vi "VMI_delays_combine.vi"(0 "Peak Array All":cluster{"X":sgl, "Y":sgl}[][][](array[cluster]), 4 "AI per delay All":dbl[][][](array[numeric]), 5 "Peak Array Current":cluster{"X":sgl, "Y":sgl}[][][](array[cluster]), 6 "AI per delay Current":dbl[][][](array[numeric]), 7 "Delay Number":i32, 9 "Counts per delay All":dbl[][][](array[numeric]), 10 "Std per delay All":dbl[][][](array[numeric]), 11 "Counts per delay Current":dbl[][][](array[numeric]), 15 "Std per delay Current":dbl[][][](array[numeric])) -> (1 "Peak Out":cluster{"X":sgl, "Y":sgl}[][][](array[cluster]), 3 "AI Out":dbl[][][](array[numeric]), 12 "Counts Out":dbl[][][](array[numeric]), 14 "Std Out":dbl[][][](array[numeric]))   [LabVIEW 2020]
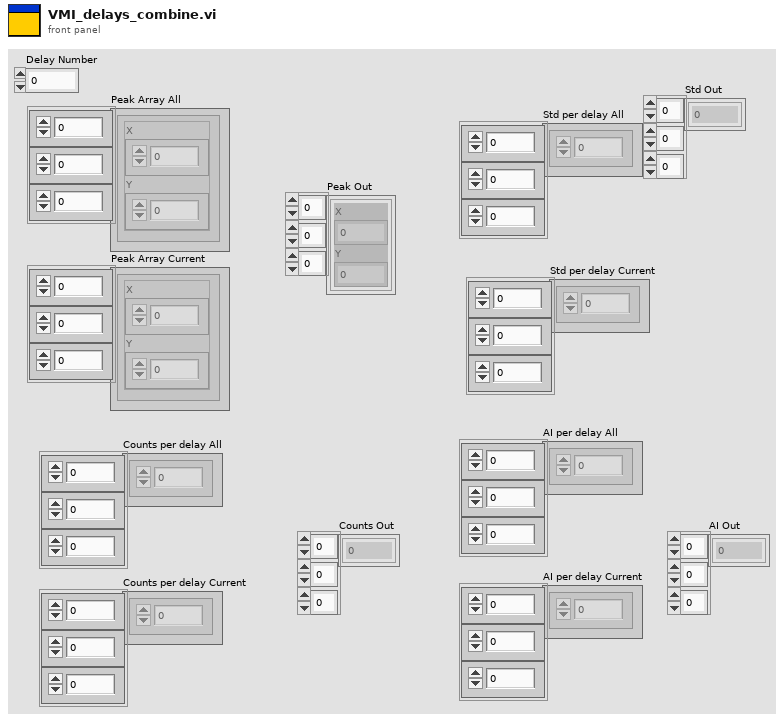
[diagram p1: front panel]
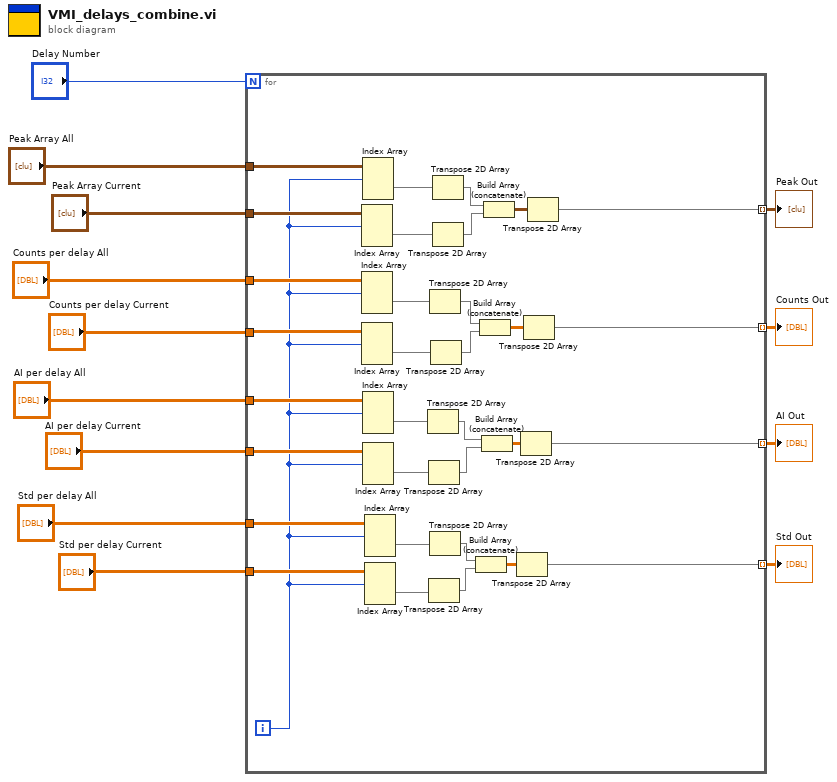
[diagram p0: block diagram]
diagram:
  n1 = for {
    N: "Delay Number" -> [_]
    tunnel: "Peak Array All" -> [w46]
    tunnel: "Counts per delay All" -> [w45]
    tunnel: "AI per delay All" -> [w44]
    tunnel: "Std per delay All" -> [w43]
    tunnel: "Peak Array Current" -> [w41]
    tunnel: [w36] -> w7 mode=indexing
    tunnel: "Counts per delay Current" -> [w34]
    tunnel: [w29] -> w5 mode=indexing
    tunnel: "AI per delay Current" -> [w28]
    tunnel: [w22] -> w3 mode=indexing
    tunnel: "Std per delay Current" -> [w21]
    tunnel: [w14] -> w1 mode=indexing
    i -> [w20]
    n2 = Index Array(array=w41, index (dim 0)=w20) -> (element=w40:cluster{"X":sgl, "Y":sgl}[][])  [unwired: 2 in]
    n3 = Index Array(array=w45, index (dim 0)=w20) -> (element=w35:dbl[][])  [unwired: 2 in]
    n4 = Index Array(array=w34, index (dim 0)=w20) -> (element=w33:dbl[][])  [unwired: 2 in]
    n5 = Index Array(array=w46, index (dim 0)=w20) -> (element=w42:cluster{"X":sgl, "Y":sgl}[][])  [unwired: 2 in]
    n6 = Index Array(array=w44, index (dim 0)=w20) -> (element=w27:dbl[][])  [unwired: 2 in]
    n7 = Index Array(array=w28, index (dim 0)=w20) -> (element=w26:dbl[][])  [unwired: 2 in]
    n8 = Index Array(array=w43, index (dim 0)=w20) -> (element=w19:dbl[][])  [unwired: 2 in]
    n9 = Index Array(array=w21, index (dim 0)=w20) -> (element=w18:dbl[][])  [unwired: 2 in]
    n10 = Transpose 2D Array(2D array=w27) -> (transposed array=w25:dbl[][])
    n11 = Transpose 2D Array(2D array=w26) -> (transposed array=w24:dbl[][])
    n12 = Transpose 2D Array(2D array=w18) -> (transposed array=w16:dbl[][])
    n13 = Transpose 2D Array(2D array=w35) -> (transposed array=w32:dbl[][])
    n14 = Transpose 2D Array(2D array=w19) -> (transposed array=w17:dbl[][])
    n15 = Transpose 2D Array(2D array=w33) -> (transposed array=w31:dbl[][])
    n16 = Transpose 2D Array(2D array=w42) -> (transposed array=w39:cluster{"X":sgl, "Y":sgl}[][])
    n17 = Transpose 2D Array(2D array=w40) -> (transposed array=w38:cluster{"X":sgl, "Y":sgl}[][])
    n18 = Build Array (concatenate)(w17, w16) -> (w15:dbl[][])
    n19 = Build Array (concatenate)(w32, w31) -> (w30:dbl[][])
    n20 = Build Array (concatenate)(w25, w24) -> (w23:dbl[][])
    n21 = Build Array (concatenate)(w39, w38) -> (w37:cluster{"X":sgl, "Y":sgl}[][])
    n22 = Transpose 2D Array(2D array=w15) -> (transposed array=w14:dbl[][])
    n23 = Transpose 2D Array(2D array=w23) -> (transposed array=w22:dbl[][])
    n24 = Transpose 2D Array(2D array=w30) -> (transposed array=w29:dbl[][])
    n25 = Transpose 2D Array(2D array=w37) -> (transposed array=w36:cluster{"X":sgl, "Y":sgl}[][])
  }
  "Peak Out" <- w7
  "Counts Out" <- w5
  "AI Out" <- w3
  "Std Out" <- w1
